vi "redovi.vi"() -> ()   [LabVIEW 2023]
uses:
  enum_typedef.ctl
panel:
  out "Enum 2":T1
  out "Numeric":i32
  in  "Enum":T1
  in  "stop":bool
  in  "Run Test 2":bool
  in  "Run Test 1":bool
  out "error out":errorcluster
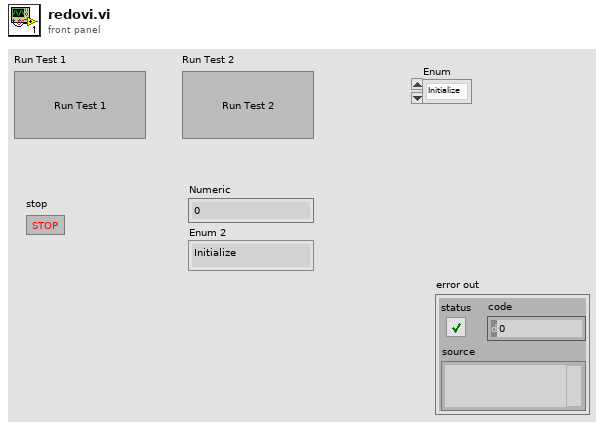
[diagram p1: front panel]
types:
  T1 = typedef "enum_typedef.ctl" = enum16{"Initialize", "Run Test 1", "Run Test 2", "Wait", "Shutdown"}
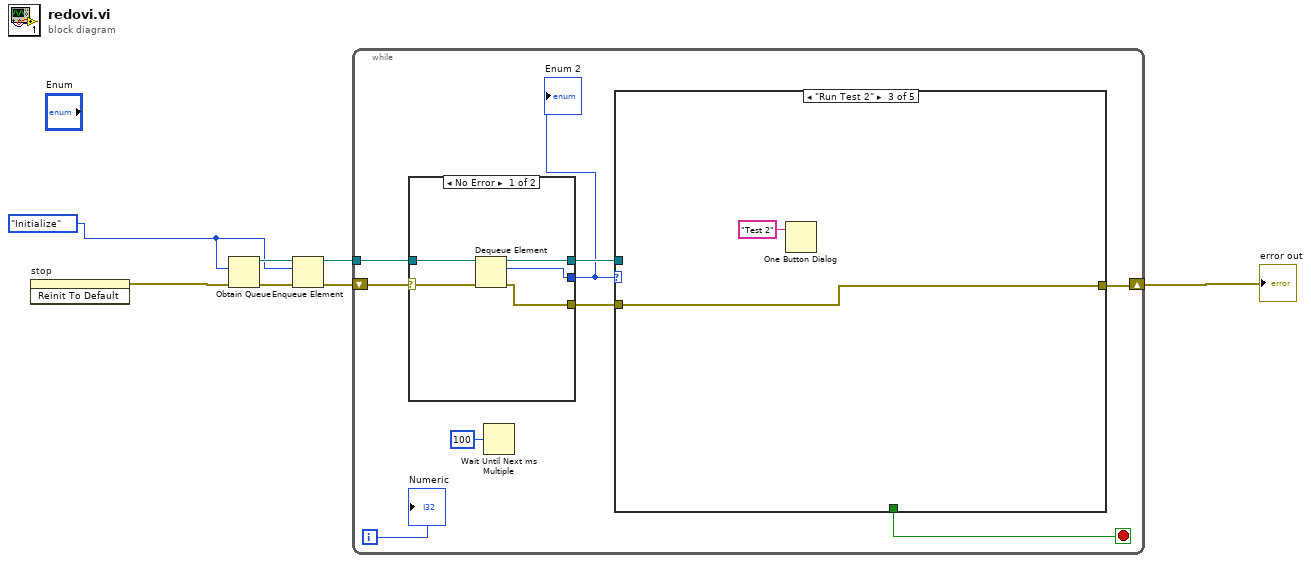
[diagram p0: block diagram]
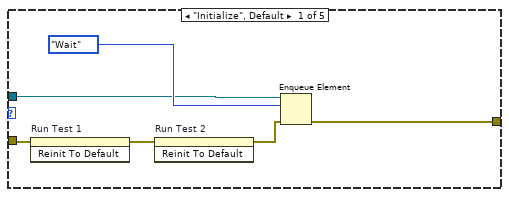
[diagram p2: hidden frame]
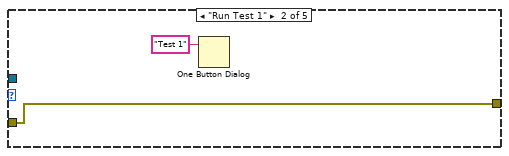
[diagram p3: hidden frame]
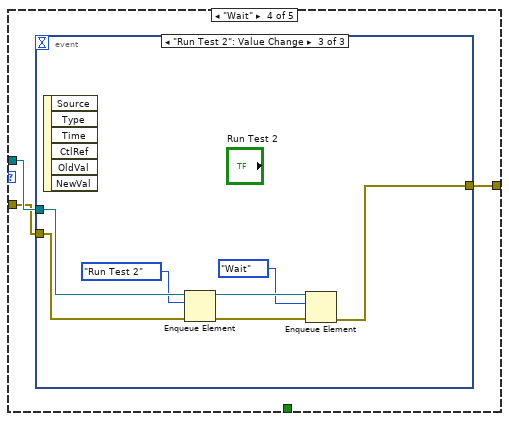
[diagram p4: hidden frame]
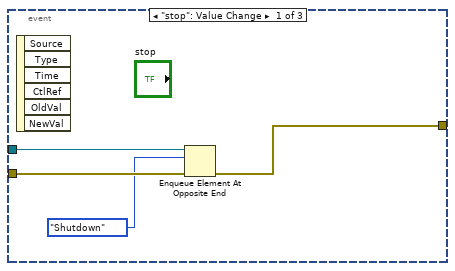
[diagram p5: hidden frame]
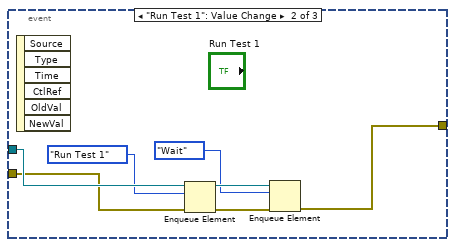
[diagram p6: hidden frame]
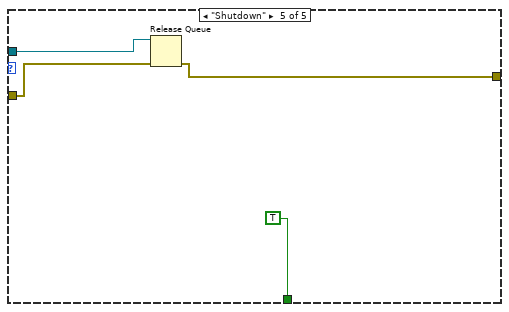
[diagram p7: hidden frame]
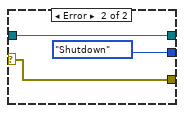
[diagram p8: hidden frame]
diagram:
  w1 = enum_typedef."Initialize" ("Enum")
  n1 = invoke on="stop" class="Bool" method="Reinit To Default"() -> (error out=w4:errorcluster)  [unwired: 3 in, 2 out]
  n2 = Obtain Queue(element data type=w1, error in (no error)=w4) -> (queue out=w3:refnum<queue>, error out=w7:errorcluster)  [unwired: 3 in, 1 out]
  n3 = Enqueue Element(queue=w3, element=w1, error in (no error)=w7) -> (queue out=w2:refnum<queue>, error out=w6:errorcluster)  [unwired: 1 in, 1 out]
  n4 = while {
    shift-right: [w11] -> w5
    shift-left: w6 -> [w16]
    tunnel: w2 -> [w15]
    i -> [w9]
    stop <- w10 stop-if-true
    n5 = case shown="No Error" w16 {
      selector: w16 -> [w56 w59]
      tunnel: w15 -> [w55 w57]
      tunnel: [w54 w57] -> w12
      tunnel: [w53 enum_typedef."Shutdown" ("Enum")] -> w8
      tunnel: [w52 w59] -> w14
      frame No Error {
        n6 = Dequeue Element(queue=w55, error in (no error)=w56) -> (queue out=w54:refnum<queue>, element=w53:T1, error out=w52:errorcluster)  [unwired: 1 in, 1 out]
      }
      frame Error {
      }
    }
    "Enum 2" <- w8
    n7 = Wait Until Next ms Multiple(millisecond multiple=u32 100) -> ()  [unwired: 1 out]
    n8 = case shown="\"Run Test 2\"" w8 {
      tunnel: w14 -> [w22 w23 w25 w28 w49]
      tunnel: w12 -> [w19 _ _ w29 w50]
      tunnel: [w17 w23 w25 w27 w48] -> w11
      tunnel: [_ _ _ _ TRUE] -> w10
      frame "Initialize", Default {
        n9 = invoke on="Run Test 1" class="Bool" method="Reinit To Default"(error in=w22) -> (error out=w21:errorcluster)  [unwired: 2 in, 2 out]
        n10 = invoke on="Run Test 2" class="Bool" method="Reinit To Default"(error in=w21) -> (error out=w18:errorcluster)  [unwired: 2 in, 2 out]
        n11 = Enqueue Element(queue=w19, element=enum_typedef."Wait" ("Enum"), error in (no error)=w18) -> (error out=w17:errorcluster)  [unwired: 1 in, 2 out]
      }
      frame "Run Test 1" {
        n12 = One Button Dialog(message="Test 1") -> ()  [unwired: 1 in, 1 out]
      }
      frame "Run Test 2" {
        n13 = One Button Dialog(message="Test 2") -> ()  [unwired: 1 in, 1 out]
      }
      frame "Wait" {
        n14 = event shown="[2] \"Run Test 2\": Value Change" {
          selector: _ -> [_ _ _]
          dyn-events: _ -> [_ _ _]
          timeout: _ -> [_ _ _]
          tunnel: w29 -> [w33 w40 w44]
          tunnel: w28 -> [w32 w36 w47]
          tunnel: [w30 w34 w45] -> w27
          event "stop": Value Change {
            n15 = event-data() -> ()  [unwired: 1 in, 6 out]
            n16 = Enqueue Element At Opposite End(queue=w33, element=enum_typedef."Shutdown" ("Enum"), error in (no error)=w32) -> (error out=w30:errorcluster)  [unwired: 1 in, 2 out]
          }
          event "Run Test 1": Value Change {
            n17 = event-data() -> ()  [unwired: 1 in, 6 out]
            n18 = Enqueue Element(queue=w40, element=enum_typedef."Run Test 1" ("Enum"), error in (no error)=w36) -> (queue out=w39:refnum<queue>, error out=w35:errorcluster)  [unwired: 1 in, 1 out]
            n19 = Enqueue Element(queue=w39, element=enum_typedef."Wait" ("Enum"), error in (no error)=w35) -> (error out=w34:errorcluster)  [unwired: 1 in, 2 out]
          }
          event "Run Test 2": Value Change {
            n20 = event-data() -> ()  [unwired: 1 in, 6 out]
            n21 = Enqueue Element(queue=w44, element=enum_typedef."Run Test 2" ("Enum"), error in (no error)=w47) -> (queue out=w43:refnum<queue>, error out=w46:errorcluster)  [unwired: 1 in, 1 out]
            n22 = Enqueue Element(queue=w43, element=enum_typedef."Wait" ("Enum"), error in (no error)=w46) -> (error out=w45:errorcluster)  [unwired: 1 in, 2 out]
          }
        }
      }
      frame "Shutdown" {
        n23 = Release Queue(queue=w50, error in (no error)=w49) -> (error out=w48:errorcluster)  [unwired: 1 in, 2 out]
      }
    }
    "Numeric" <- w9
  }
  "error out" <- w5
